vi "RSZVB Configure Port PI Controller.vi"(5 "Integration Time (500.0E-9)":dbl=5e-07 format="%^.3e", 6 "Gain (0.4)":dbl=0.4 format="%^.3e", 7 "PI Controller Mode (Auto)":i32(ring) items=["Auto", "Manual"], 8 "error in (no error)":errorcluster {"code" format="%.0x"}, 9 "Port (1)":i32=1, 10 "Channel (1)":i32=1, 11 "VISA session":refnum<visa-resource-name>) -> (0 "error out":errorcluster {"code" format="%.0x"}, 3 "dup VISA session":refnum<visa-resource-name>)   [LabVIEW 2011]
doc: "Configures PI controller parameters at source port <Pt>. \n\nRemote-control command(s):\nSOURce<Ch>:POWer<Pt>:ALC:PIParameter\nSOURce<Ch>:POWer<Pt>:ALC:PIParameter:GAIN\nSOURce<Ch>:POWer<Pt>:ALC:PIParameter:ITIMe"
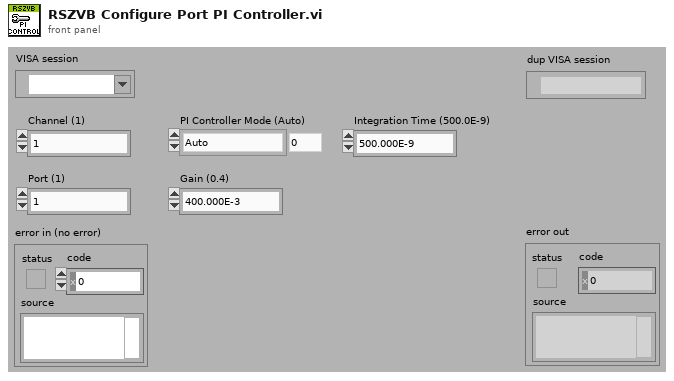
[diagram p1: front panel]
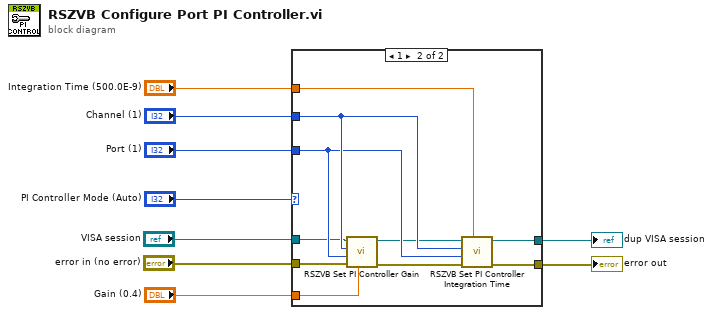
[diagram p0: block diagram]
diagram:
  n1 = case shown="1" "PI Controller Mode (Auto)" {
    tunnel: "Channel (1)" -> [_ w19]
    tunnel: "Port (1)" -> [_ w18]
    tunnel: "Gain (0.4)" -> [_ w21]
    tunnel: "Integration Time (500.0E-9)" -> [_ w20]
    tunnel: "VISA session" -> [w11 w17]
    tunnel: "error in (no error)" -> [w10 w16]
    tunnel: [w11 w13] -> w2
    tunnel: [w10 w12] -> w1
    frame 0, Default {
    }
    frame 1 {
      n2 = call "RSZVB Set PI Controller Gain.vi"("Gain (0.4)"=w21, "error in (no error)"=w16, "Port (1)"=w18, "Channel (1)"=w19, "VISA session"=w17) -> ("error out"=w14:errorcluster, "dup VISA session"=w15:refnum<visa-resource-name>)  [unwired: 5 in]
      n3 = call "RSZVB Set PI Controller Integration Time.vi"("Integration Time (500.0E-9)"=w20, "error in (no error)"=w14, "Port (1)"=w18, "Channel (1)"=w19, "VISA session"=w15) -> ("error out"=w12:errorcluster, "dup VISA session"=w13:refnum<visa-resource-name>)  [unwired: 5 in]
    }
  }
  "error out" <- w1
  "dup VISA session" <- w2
